vi "Parse Waveform from Result.vi"(8 "error in (no error)":errorcluster, 11 "ReadCommand":refnum<class "ReadCommand.lvclass">) -> (0 "error out":errorcluster, 3 "Waveform":waveform(dbl)[](array[waveform]))   [LabVIEW 2023]
uses:
  Measure/Measure.lvclass
  Parameter/Parameter.lvclass
  HAF.lvlib
  ReadCommand/ReadCommand.lvclass
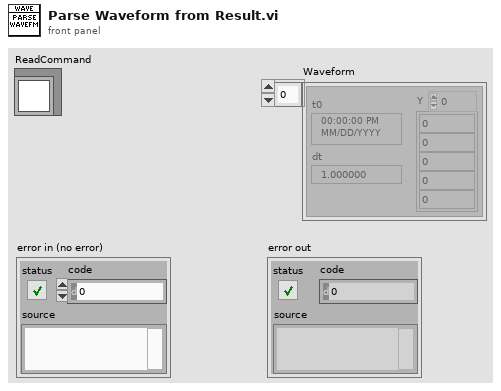
[diagram p1: front panel]
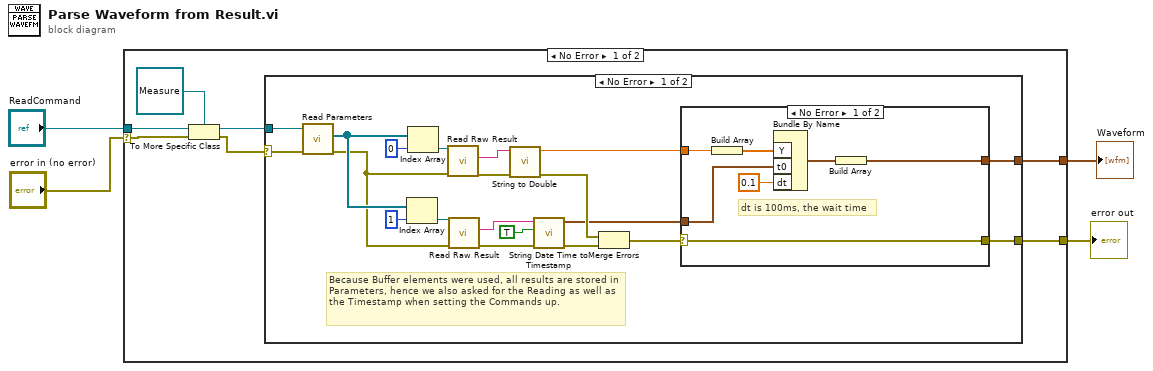
[diagram p0: block diagram]
diagram:
  n1 = case shown="No Error" "error in (no error)" {
    selector: "error in (no error)" -> [w9 w41]
    tunnel: "ReadCommand" -> [w10 _]
    tunnel: [w6 _] -> w2
    tunnel: [w5 w41] -> w1
    frame No Error {
      n2 = To More Specific Class(target class=refnum<class "Measure.lvclass"> refnum ("HAF:Measure.lvclass"), reference=w10, error in=w9) -> (specific class reference=w7:refnum<class "Measure.lvclass">, error out=w8:errorcluster)
      n3 = case shown="No Error" w8 {
        selector: w8 -> [w30 w40]
        tunnel: w7 -> [w31 _]
        tunnel: [w13 _] -> w6
        tunnel: [w12 w40] -> w5
        frame No Error {
          # "Because Buffer elements were used, all results are stored in Parameters, hence we also asked for the Reading as well as the Timestamp when setting the Commands up."
          n4 = call-dynamic "Read Parameters.vi"("error in (no error)"=w30, "WriteCommand in"=w31) -> ("error out"=w22:errorcluster, "Parameters"=w28:refnum<class "Parameter.lvclass">[])  [unwired: 7 in, 1 out]
          n5 = Index Array(array=w28, index=1) -> (element=w23:refnum<class "Parameter.lvclass">)
          n6 = Index Array(array=w28, index=0) -> (element=w26:refnum<class "Parameter.lvclass">)
          n7 = call-dynamic "Read Raw Result.vi"("error in (no error)"=w22, "Parameter in"=w26) -> ("error out"=w24:errorcluster, "Raw Result"=w25:string)  [unwired: 7 in, 1 out]
          n8 = call-dynamic "Read Raw Result.vi"("error in (no error)"=w22, "Parameter in"=w23) -> ("error out"=w20:errorcluster, "Raw Result"=w21:string)  [unwired: 7 in, 1 out]
          n9 = call "String to Double.vi"("error in (no error)"=w24, "String to Convert"=w25) -> ("error out"=w17:errorcluster, "Double Value"=w15:dbl)  [unwired: 8 in]
          n10 = call "String Date Time to Timestamp.vi"("error in (no error)"=w20, "Use milliseconds"=TRUE, "String to Convert"=w21) -> ("error out"=w18:errorcluster, "Timestamp Value"=w14:timestamp)  [unwired: 7 in]
          n11 = Merge Errors(w17, w18) -> (w16:errorcluster)
          n12 = case shown="No Error" w16 {
            selector: w16 -> [w32 w39]
            tunnel: w15 -> [w38 _]
            tunnel: w14 -> [w36 _]
            tunnel: [w33 _] -> w13
            tunnel: [w32 w39] -> w12
            frame No Error {
              # "dt is 100ms, the wait time"
              n13 = Build Array(w38) -> (w37:dbl[])
              n14 = Bundle By Name("Y"=w37, "t0"=w36, "dt"=0.1) -> (w34:waveform(dbl))  [unwired: 1 in]
              n15 = Build Array(w34) -> (w33:waveform(dbl)[])
            }
            frame Error {
            }
          }
        }
        frame Error {
        }
      }
    }
    frame Error {
    }
  }
  "error out" <- w1
  "Waveform" <- w2
